vi "Create.vi"() -> (0 "error out":errorcluster, 3 "CloneRegRef":refnum<data-value>)   [LabVIEW 2014, in "ModuleAdmin.lvlib" / "CloneRegistration.lvclass"]
uses:
  CloneRegistration.lvclass
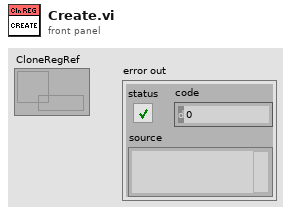
[diagram p1: front panel]
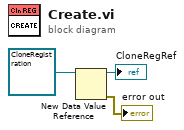
[diagram p0: block diagram]
diagram:
  n1 = New Data Value Reference(data value=refnum<class "CloneRegistration.lvclass"> refnum ("NistModuleAdmin.lvlib:CloneRegistration.lvclass")) -> (data value reference=→"CloneRegRef":refnum<data-value>, error out=→"error out":errorcluster)  [unwired: 1 in]
